vi "Chroma load current change.vi"() -> ()   [LabVIEW 2011]
uses:
  instr.lib/Chroma 63600/Chroma 63600.lvlib
panel:
  in  "Channel":i8=1 min=1 max=10
  in  "error in (no error)":errorcluster
  in  "value":dbl
  in  "VISA resource name":refnum<visa-resource-name>="GPIB0::7::INSTR"
  out "VISA resource name out":refnum<visa-resource-name>
  out "error out":errorcluster
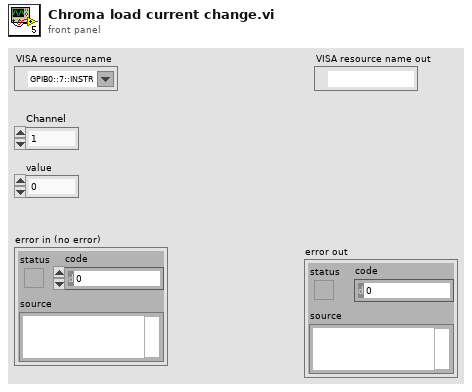
[diagram p1: front panel]
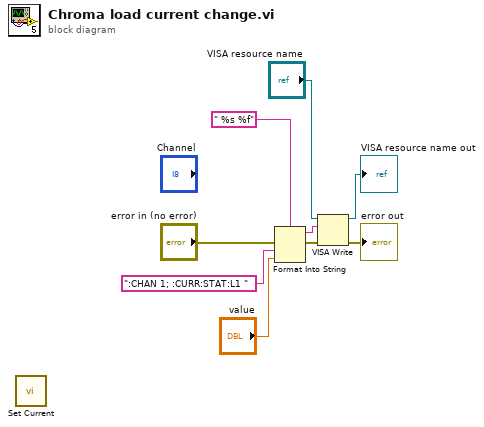
[diagram p0: block diagram]
diagram:
  n1 = call "Set Current.vi"() -> ()  [unwired: 10 in, 2 out]
  n2 = Format Into String(format string=" %s %f", error in="error in (no error)", ":CHAN 1; :CURR:STAT:L1 " ("input 2"), "value") -> (resulting string=w5:string, error out=w4:errorcluster)  [unwired: 1 in]
  n3 = VISA Write(VISA resource name="VISA resource name", write buffer=w5, error in (no error)=w4) -> (VISA resource name out=→"VISA resource name out":refnum<visa-resource-name>, error out=→"error out":errorcluster)  [unwired: 1 out]
